vi "frequency_write.vi"() -> ()   [LabVIEW 2018]
uses:
  <vilib>/rvi/FXPMathLib/FxpDiv/subVIs/nifxpmath_Div_SimConfig.ctl
  <vilib>/rvi/FXPMathLib/FxpDiv/simVIs/DllFxpDivTemp_sub.vi
  <vilib>/rvi/Memory/Memory_Emulation/nirvimemoryFastEmulation.vi
  <vilib>/rvi/Memory/Memory_Emulation/nirvimemoryEmulation.vi
  <vilib>/rvi/Emulation/niFpgaEmulationIsFPGAContextNoSignature.vi
  <vilib>/rvi/DataTransferAndStorage/Container/Common/niFpgaContainerGetUniqueNameForEmu.vi
  <vilib>/rvi/Emulation/niFpgaProcessEmulError.vi
  <vilib>/rvi/Emulation/niFpgaSctlEmulationGetInTimedLoop.vi
  <vilib>/rvi/errors/nirviReportUnexpectedCaseInternalError (U32).vi
  <vilib>/rvi/FXPMathLib/FxpDiv/XNode/nifxpmath_Div.xnode
  <vilib>/rvi/DataTransferAndStorage/Container/XNode/niFpgaContainer.xnode
panel:
  out "frequency_actual":u32
  in  "index":u8
  in  "frequency_requested":u32
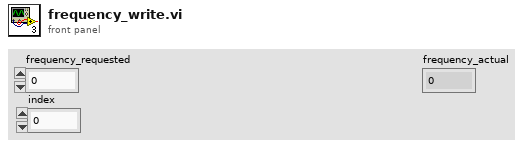
[diagram p1: front panel]
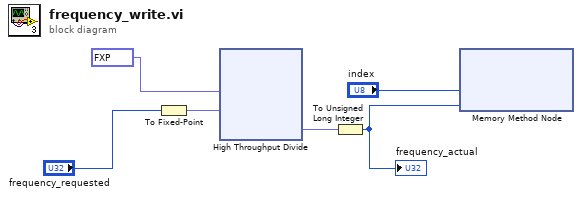
[diagram p0: block diagram]
diagram:
  n1 = To Fixed-Point(number="frequency_requested") -> (fixed-point=w6:fxp<+,18,18>)  [unwired: 1 in]
  n2 = xnode "High Throughput Divide"("x"=fxp<+,17,18> 156250.0, "y"=w6) -> ("x/y"=w4:fxp<+,18,18>)
  n3 = To Unsigned Long Integer(number=w4) -> (unsigned 32bit integer=w2:u32)
  "frequency_actual" <- w2
  n4 = xnode ("Memory Method Node")("Address"="index", "Data"=w2) -> ()  [unwired: 1 in, 1 out]
